vi "Main.vi"(8 "Error In":errorcluster, 11 "Simulate hardware?":bool) -> (0 "Error Out":errorcluster)   [LabVIEW 2017, in "DAQ.lvlib"]
uses:
  DAQ.lvlib
  Controls/Commands [enum].ctl
  Controls/Params.ctl
  Controls/DAQ Config.ctl
  Controls/DAQ Indicators.ctl
  System Control/CTLs/Test Type.ctl
  File IO/Controls/Params.ctl
  Events/Controls/Action Refs [enum].ctl
  Background Level Global.vi
  System Control/Main controller.lvlib
  Events/Events.lvlib
  File IO/File IO.lvlib
  UI/UI.lvlib
panel:
  out "Indicators":T1={"Data"={"Live"={"t0"=timestamp(0 s since 1904-01-01), "dt"=1.0, "Y"=[]}, "Accumulated"={"t0"=timestamp(0 s since 1904-01-01), "dt"=1.0, "Y"=[]}, "Averaged"={"t0"=timestamp(0 s since 1904-01-01), "dt"=1.0, "Y"=[]}, "data array"=[], "live time array"=[], "Live (decimated)"={"t0"=timestamp(0 s since 1904-01-01), "dt"=1.0, "Y"=[]}}, "Config"={"Input Config"=-1, "Card"=enum."USB-6211", "100% Reflectance Standard (V)"=1.0, "Input Channel"="", "Average number of points"=50.0, "Trigger Level (V)"=0.2, "Rate (Hz)"=250000, "End Time (s)"=1.0}, "Indicators"={"Final number of points"=5500.0, "Number of samples"=275000.0, "dt"=4e-06, "Shots"=1, "Shot counter"=0, "Test counter"=0, "Background level (V)"=0.0, "DAQ task"="", "timestamp of data"=timestamp(0 s since 1904-01-01), "Test Type"=enum."A-Test"}} {"Config"."Input Config" items=["default"=-1, "RSE"=10083, "NRSE"=10078, "Differential"=10106, "Pseudodifferential"=12529]}
  in  "File IO parameters - DEBUG":T5={"Output Folder"=path "C:/Users/Abigail/Documents/Imperial Optical software/Optical Software Code Simplified/Output", "Error file"=path "Error Log.txt", "Config file"=path "Config.ini", "File prefix"="600 nm", "Waveform read"={"t0"=timestamp(0 s since 1904-01-01), "dt"=1.0, "Y"=[]}}
  out "Live data incl. pre-trigger":cluster{"live time array":dbl[], "Y":dbl[]}(graph)
  out "Live data (cropped)":dbl[](graph)
  out "Accumulated data":waveform(dbl)(graph)={"t0"=timestamp(3604915966.0623617 s since 1904-01-01), "dt"=0.00019999999999999998, "Y"=[]}
  out "Averaged data":waveform(dbl)(graph)={"t0"=timestamp(3604915977.982374 s since 1904-01-01), "dt"=0.00019999999999999998, "Y"=[]}
  in  "Config In":T1={"Data"={"Live"={"t0"=timestamp(0 s since 1904-01-01), "dt"=1.0, "Y"=[]}, "Accumulated"={"t0"=timestamp(0 s since 1904-01-01), "dt"=1.0, "Y"=[]}, "Averaged"={"t0"=timestamp(0 s since 1904-01-01), "dt"=1.0, "Y"=[]}, "data array"=[], "live time array"=[], "Live (decimated)"={"t0"=timestamp(0 s since 1904-01-01), "dt"=1.0, "Y"=[]}}, "Config"={"Input Config"=-1, "Card"=enum."USB-6211", "100% Reflectance Standard (V)"=1.0, "Input Channel"="", "Average number of points"=50.0, "Trigger Level (V)"=0.2, "Rate (Hz)"=250000, "End Time (s)"=1.0}, "Indicators"={"Final number of points"=5500.0, "Number of samples"=275000.0, "dt"=4e-06, "Shots"=1, "Shot counter"=0, "Test counter"=0, "Background level (V)"=0.0, "DAQ task"="", "timestamp of data"=timestamp(0 s since 1904-01-01), "Test Type"=enum."A-Test"}} {"Config"."Input Config" items=["default"=-1, "RSE"=10083, "NRSE"=10078, "Differential"=10106, "Pseudodifferential"=12529]}
  in  "Set state":T6
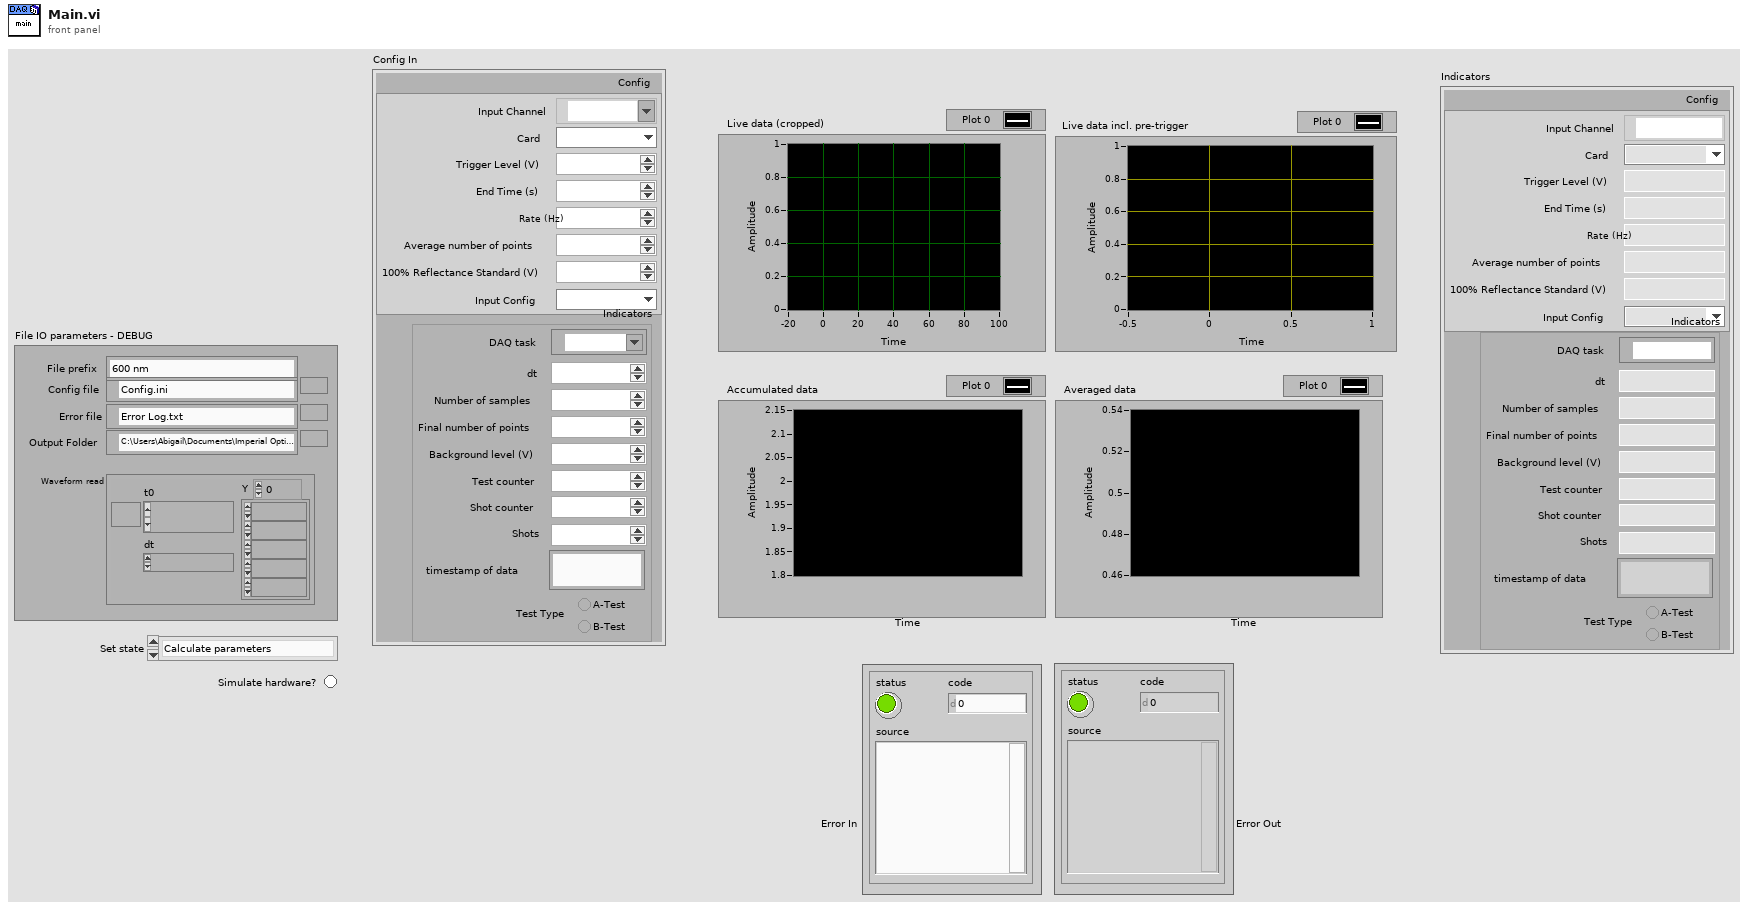
[diagram p1: front panel]
types:
  T1 = typedef "DAQ.lvlib/Params.ctl" = cluster{"Data":cluster{"Live":waveform(dbl), "Accumulated":waveform(dbl), "Averaged":waveform(dbl), "data array":dbl[], "live time array":dbl[], "Live (decimated)":waveform(dbl)}, "Config":T2, "Indicators":T3}
  T2 = typedef "DAQ.lvlib/DAQ Config.ctl" = cluster{"Input Config":i32, "Card":enum16{"USB-6211", "USB-6251", "USB-6361"}, "100% Reflectance Standard (V)":dbl, "Input Channel":tag, "Average number of points":dbl, "Trigger Level (V)":dbl, "Rate (Hz)":i32, "End Time (s)":dbl}
  T3 = typedef "DAQ.lvlib/DAQ Indicators.ctl" = cluster{"Final number of points":dbl, "Number of samples":dbl, "dt":dbl, "Shots":i32, "Shot counter":i32, "Test counter":i32, "Background level (V)":dbl, "DAQ task":refnum<k21>, "timestamp of data":timestamp, "Test Type":T4}
  T4 = typedef "Main controller.lvlib/Test Type.ctl" = enum32{"A-Test", "B-Test"}
  T5 = typedef "File IO.lvlib/Params.ctl" = cluster{"Output Folder":path, "Error file":path, "Config file":path, "File prefix":string, "Waveform read":waveform(dbl)}
  T6 = typedef "DAQ.lvlib/Commands [enum].ctl" = enum16{"Calculate parameters", "Start", "Stop", "Get test data", "Accumulate test data", "Average test data", "Calculate background voltage", "Send data", "Write data to file"}
  T7 = enum32{"Bad", "Idle", "Run top level", "Running"}
  T8 = typedef "Events.lvlib/Action Refs [enum].ctl" = enum16{"Init", "Ref", "Kill"}
  T9 = typedef "Events.lvlib/Refs [cluster].ctl" = cluster{"Exit":refnum<user-event>, "Controller":refnum<user-event>, "System Error":refnum<user-event>, "UI":refnum<user-event>, "Example Module":refnum<user-event>, "Shutter":refnum<user-event>, "Monochromator":refnum<user-event>, "DAQ":refnum<user-event>, "Scope":refnum<user-event>, "Processing":refnum<user-event>, "File IO":refnum<user-event>, "Colour wheel":refnum<user-event>}
  T10 = cluster{"Live":waveform(dbl), "Accumulated":waveform(dbl), "Averaged":waveform(dbl), "data array":dbl[], "live time array":dbl[], "Live (decimated)":waveform(dbl)}
  T11 = cluster{"Waveform Data":dbl[][], "Waveform Name":string}
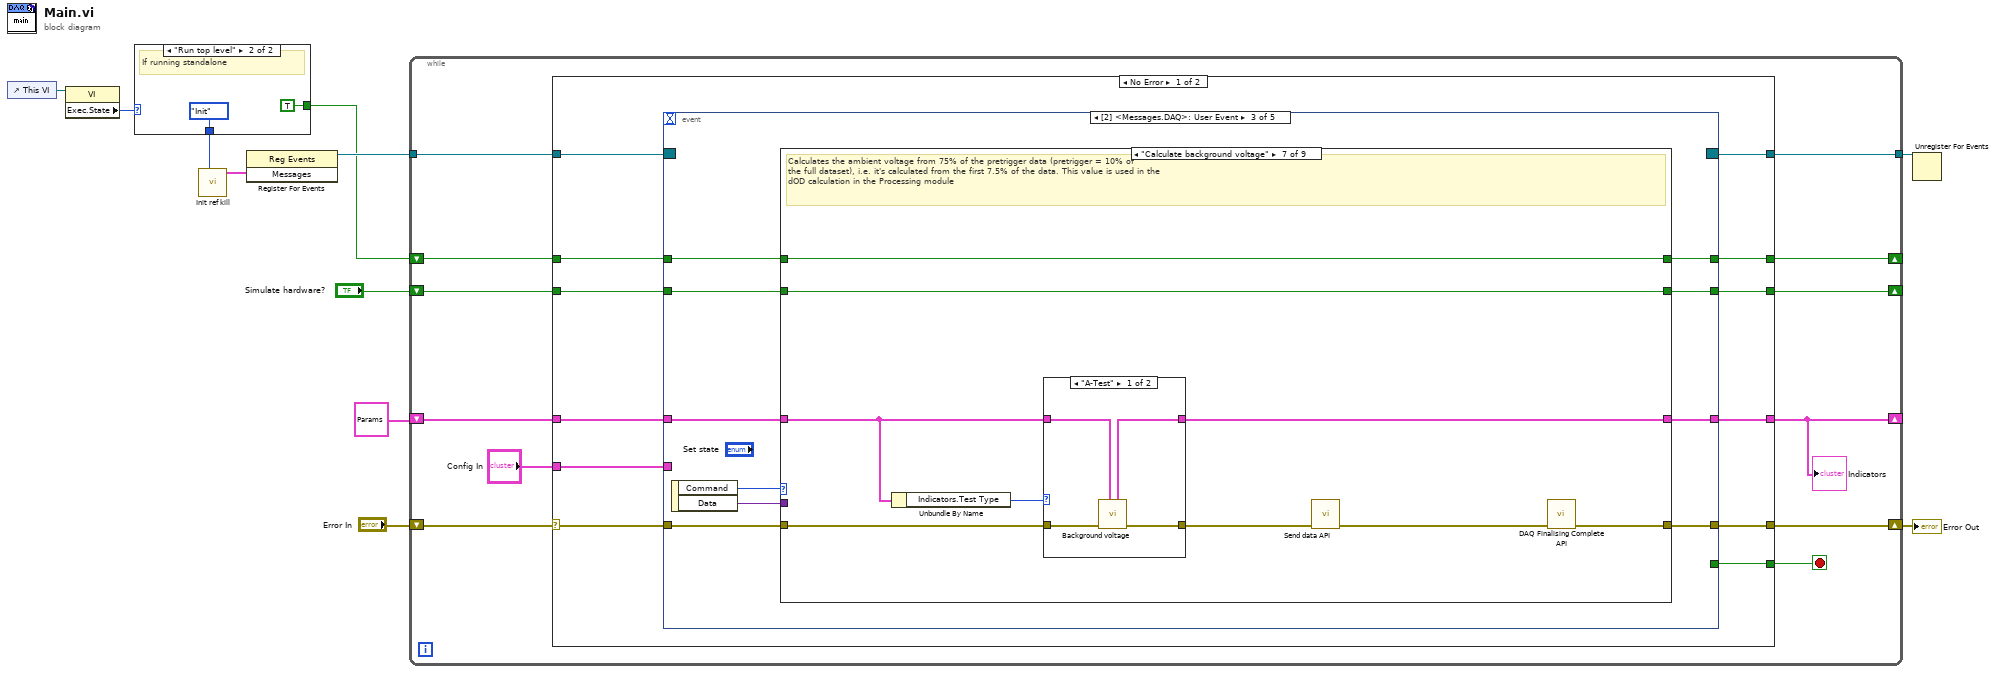
[diagram p0: block diagram]
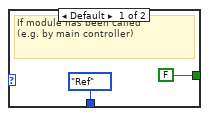
[diagram p2: hidden frame]
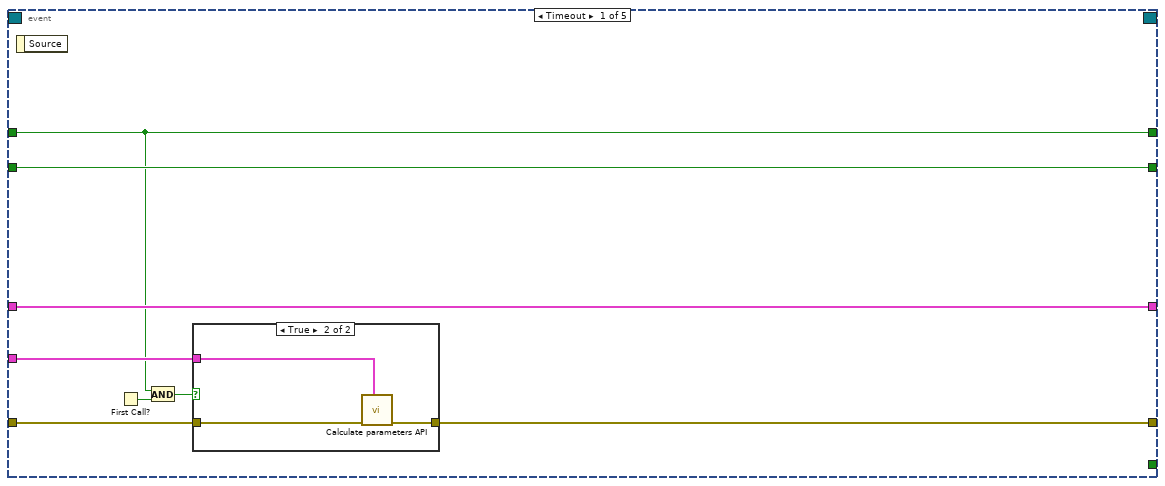
[diagram p3: hidden frame]
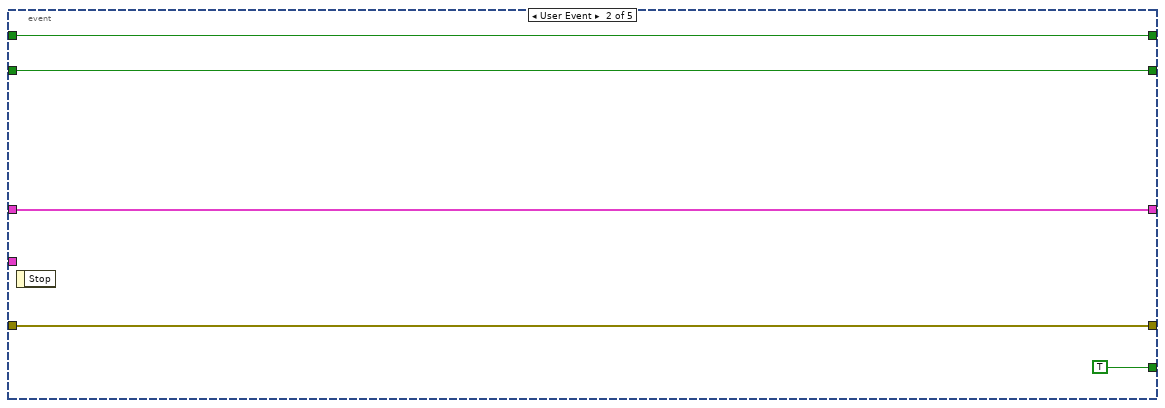
[diagram p5: hidden frame]
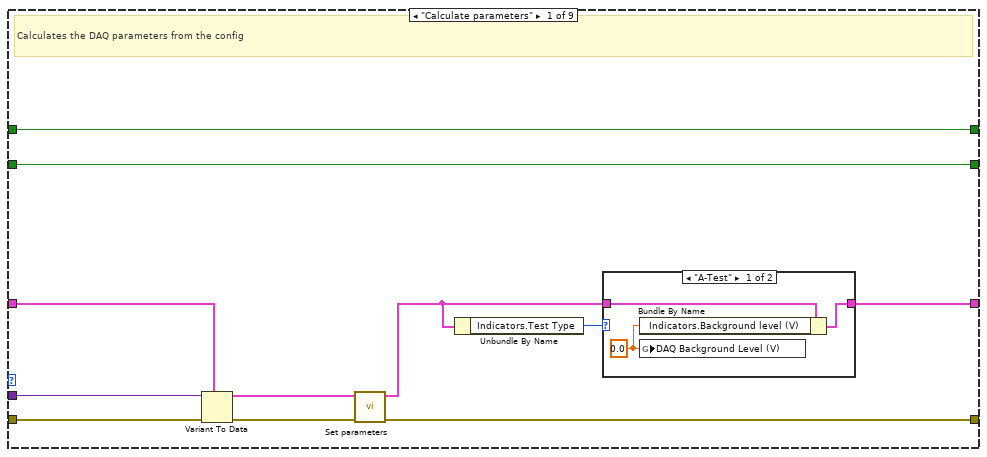
[diagram p6: hidden frame]
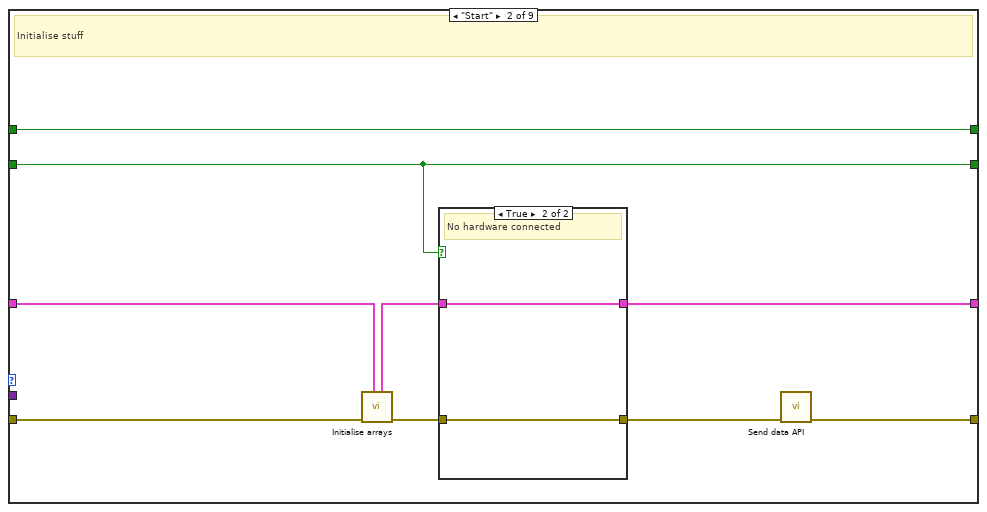
[diagram p8: hidden frame]
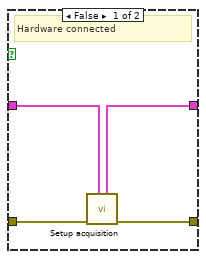
[diagram p9: hidden frame]
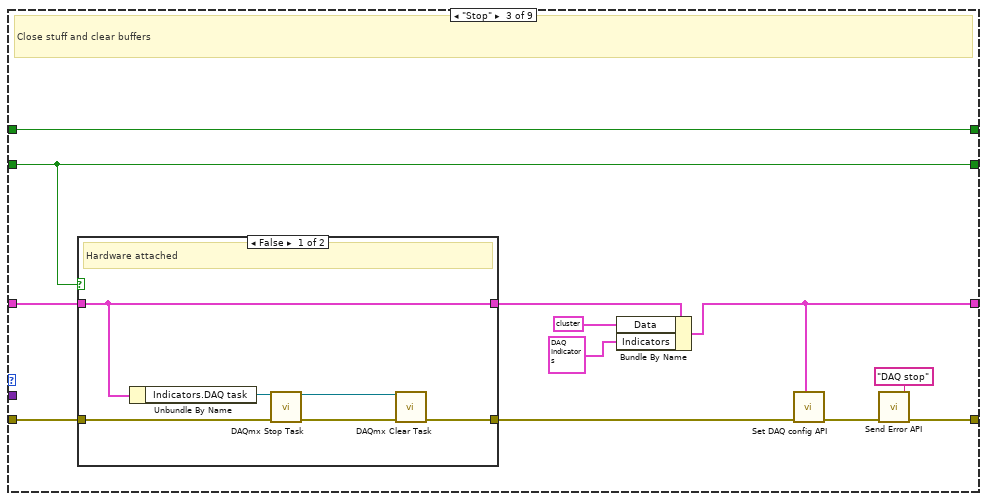
[diagram p10: hidden frame]
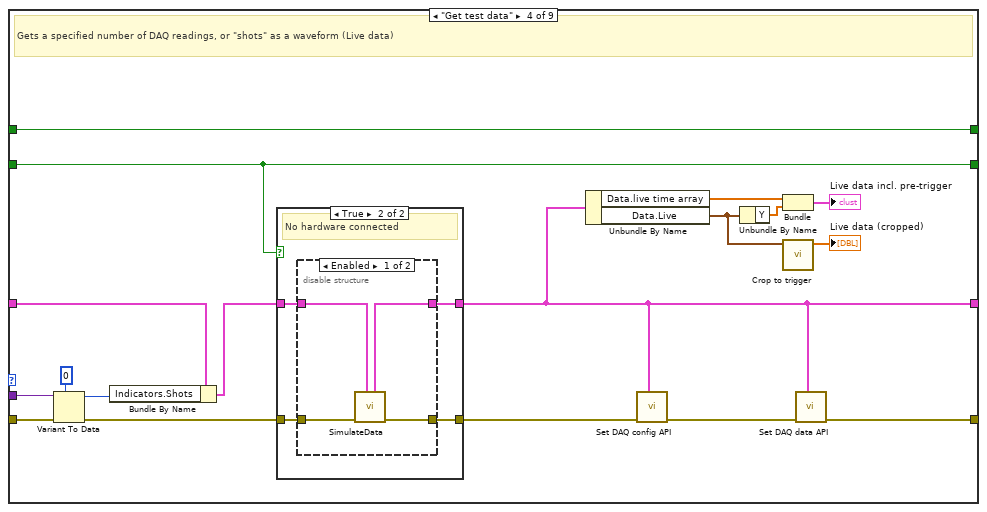
[diagram p12: hidden frame]
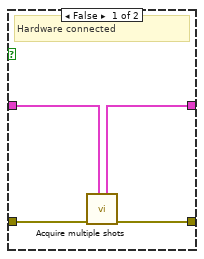
[diagram p13: hidden frame]
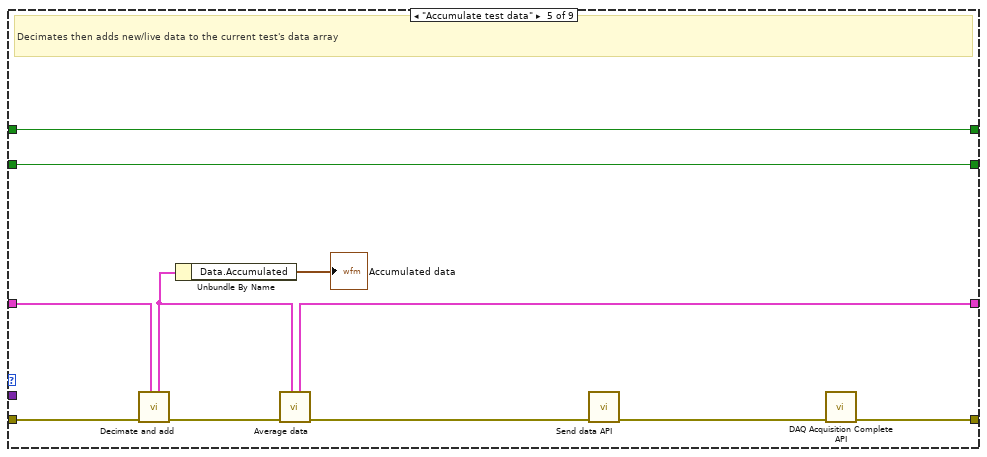
[diagram p15: hidden frame]
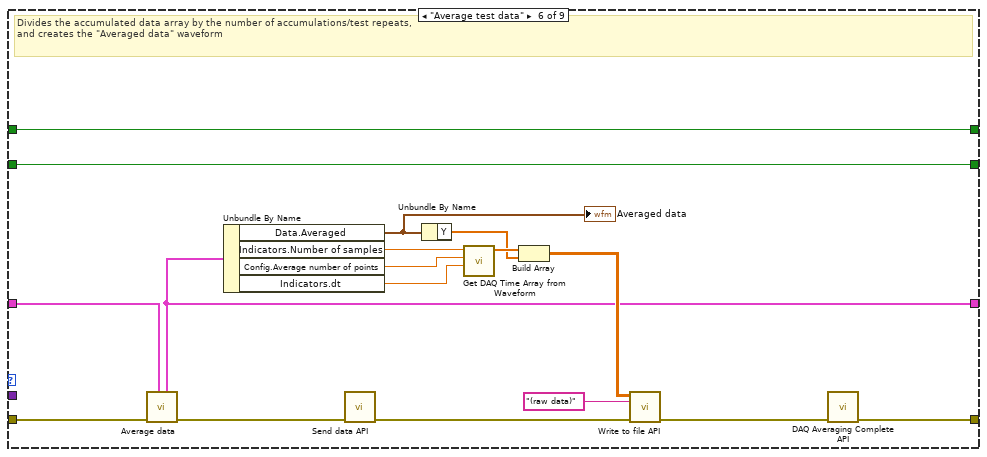
[diagram p16: hidden frame]
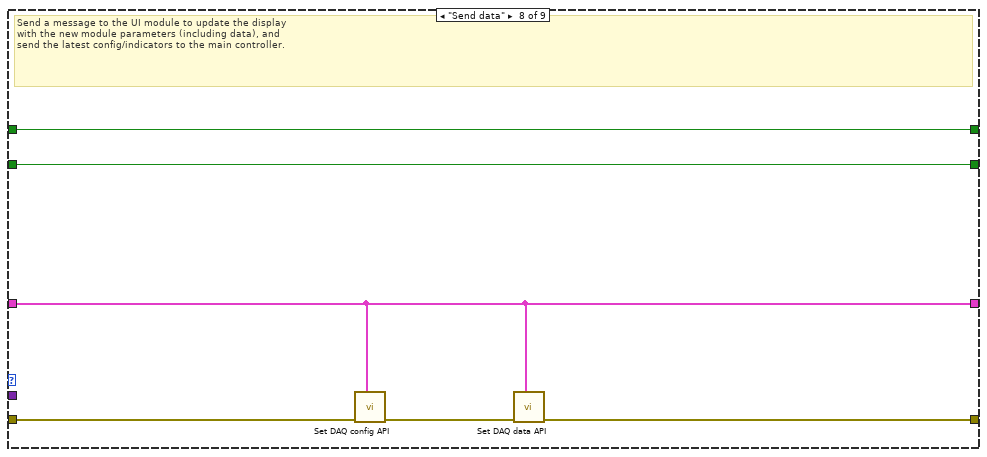
[diagram p18: hidden frame]
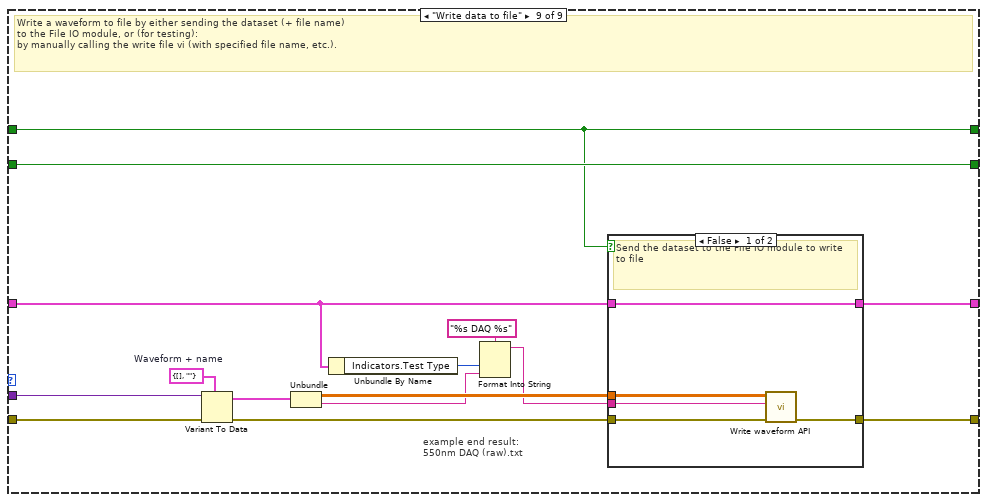
[diagram p19: hidden frame]
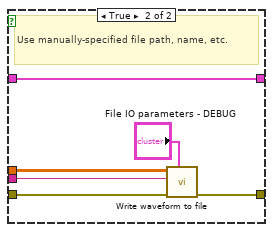
[diagram p20: hidden frame]
diagram:
  n1 = control-ref of="This VI"() -> (w6:refnum<vi>)
  n2 = property class="VI"(reference=w6) -> ("Exec.State"=w5:T7)  [unwired: 1 in, 2 out]
  n3 = case shown="\"Run top level\"" w5 {
    tunnel: [Action_Refs_[enum]."Ref" ("Action") Action_Refs_[enum]."Init" ("Action")] -> w4
    tunnel: [FALSE TRUE] -> w3
    frame Default {
      # "If module has been called\n(e.g. by main controller)"
    }
    frame "Run top level" {
      # "If running standalone"
    }
  }
  n4 = call "Init ref kill.vi"("Action"=w4) -> ("Messages"=w11:T9)  [unwired: 9 in, 1 out]
  n5 = register-events(w11) -> (reference out=w10:refnum<event-registration>)  [unwired: 2 in, 1 out]
  n6 = while {
    tunnel: w10 -> [w27]
    shift-right: [w24] -> _
    shift-left: "Simulate hardware?" -> [w23]
    tunnel: [w25] -> w9
    shift-right: [w21] -> w7
    shift-left: "Error In" -> [w20]
    shift-right: [w16] -> _
    shift-left: T1 {"Data"={"Live"={"t0"=timestamp(0 s since 1904-01-01), "dt"=1.0, "Y"=[]}, "Accumulated"={"t0"=timestamp(0 s since 1904-01-01), "dt"=1.0, "Y"=[]}, "Averaged"={"t0"=timestamp(0 s since 1904-01-01), "dt"=1.0, "Y"=[]}, "data array"=[], "live time array"=[], "Live (decimated)"={"t0"=timestamp(0 s since 1904-01-01), "dt"=1.0, "Y"=[]}}, "Config"={"Input Config"=-1, "Card"=enum."USB-6211", "100% Reflectance Standard (V)"=1.0, "Input Channel"="", "Average number of points"=50.0, "Trigger Level (V)"=0.2, "Rate (Hz)"=250000, "End Time (s)"=1.0}, "Indicators"={"Final number of points"=0.0, "Number of samples"=0.0, "dt"=0.0, "Shots"=1, "Shot counter"=0, "Test counter"=0, "Background level (V)"=0.0, "DAQ task"="", "timestamp of data"=timestamp(0 s since 1904-01-01), "Test Type"=enum."A-Test"}} ("Config 2") -> [w22]
    shift-right: [w18] -> _
    shift-left: w3 -> [w19]
    stop <- w26 stop-if-true
    n7 = case shown="No Error" w20 {
      selector: w20 -> [w31 w277]
      tunnel: w27 -> [w39 w273]
      tunnel: [w38 _] -> w26
      tunnel: [w37 w273] -> w25
      tunnel: [w36 w275] -> w24
      tunnel: w23 -> [w35 w275]
      tunnel: w22 -> [w34 w272]
      tunnel: [w33 w272] -> w16
      tunnel: [w32 w276] -> w21
      tunnel: w19 -> [w30 w274]
      tunnel: [w29 w274] -> w18
      tunnel: "Config In" -> [w28 _]
      frame No Error {
        n8 = event shown="[2] <Messages.DAQ>: User Event" {
          selector: w39 -> [_ _ _ _ _]
          dyn-events: [_ _ _ _ _] -> w37
          timeout: _ -> [_ _ _ _ _]
          tunnel: [_ TRUE _ _ _] -> w38
          tunnel: [w47 w53 w65 w228 w235] -> w36
          tunnel: w35 -> [w47 w53 w64 w228 w235]
          tunnel: w31 -> [w46 w54 w62 w226 w231]
          tunnel: [w45 w54 w61 w225 w230] -> w32
          tunnel: w34 -> [w44 w55 w60 _ w233]
          tunnel: [w44 w55 w59 w224 w232] -> w33
          tunnel: w30 -> [w42 w52 w57 w227 w229]
          tunnel: [w42 w52 w58 w227 w229] -> w29
          tunnel: w28 -> [w43 _ _ _ _]
          event Timeout {
            n9 = event-data() -> ()  [unwired: 1 in, 1 out]
            n10 = First Call?() -> (First Call?: T/F=w41:bool)
            n11 = And(x=w42, y=w41) -> (x .and. y?=w40:bool)
            n12 = case shown="True" w40 {
              tunnel: w46 -> [w48 w51]
              tunnel: [w48 w50] -> w45
              tunnel: w43 -> [_ w49]
              frame False {
              }
              frame True {
                n13 = call "Calculate parameters API.vi"("DAQ"=w49, "Error In"=w51) -> ("Error Out"=w50:errorcluster)  [unwired: 9 in]
              }
            }
          }
          event User Event {
            n14 = event-data() -> ()  [unwired: 1 in, 1 out]
          }
          event User Event {
            n15 = event-data() -> ("Command"=w66:T6, "Data"=w63:variant)  [unwired: 1 in]
            n16 = case shown="\"Calculate background voltage\"" w66 {
              tunnel: [w72 w89 w103 w131 w158 w175 w185 w197 w212] -> w65
              tunnel: w64 -> [w72 w89 w103 w131 w158 w175 w185 w197 w212]
              tunnel: w63 -> [w76 _ _ w125 _ _ _ _ w206]
              tunnel: w62 -> [w77 w86 w104 w127 w159 w176 w184 w196 w207]
              tunnel: [w71 w82 w108 w118 w154 w169 w182 w192 w203] -> w61
              tunnel: w60 -> [w75 w85 w105 w123 w155 w171 w178 w193 w200]
              tunnel: [w69 w84 w97 w117 w149 w162 w181 w193 w204] -> w59
              tunnel: [w73 w90 w106 w132 w157 w174 w183 w194 w205] -> w58
              tunnel: w57 -> [w73 w90 w106 w132 w157 w174 w183 w194 w205]
              frame "Calculate parameters" {
                # "Calculates the DAQ parameters from the config"
                n17 = Variant To Data(error in=w77, type=w75, Variant=w76) -> (data=w70:T1, error out=w74:errorcluster)
                n18 = call "Set parameters.vi"("error in"=w74, "DAQ"=w70) -> ("error out"=w71:errorcluster, "DAQ out"=w68:T1)  [unwired: 8 in]
                n19 = Unbundle By Name(w68) -> ("Indicators.Test Type"=w67:T4)
                n20 = case shown="\"A-Test\"" w67 {
                  tunnel: w68 -> [w80 w81]
                  tunnel: [w79 w81] -> w69
                  frame "A-Test" {
                    w78 = 0.0 ("DAQ Background Level (V)")
                    n21 = Bundle By Name(cluster=w80, "Indicators.Background level (V)"=w78) -> (w79:T1)
                    n22 = global write "Background Level Global.vi" "DAQ Background Level (V)"(w78) -> ()
                  }
                  frame "B-Test" {
                  }
                }
              }
              frame "Start" {
                # "Initialise stuff"
                n23 = call "Initialise arrays.vi"("DAQ"=w85, "error in"=w86) -> ("error out"=w88:errorcluster, "DAQ out"=w87:T1)  [unwired: 8 in]
                n24 = case shown="True" w89 {
                  tunnel: w88 -> [w94 w96]
                  tunnel: [w93 w96] -> w83
                  tunnel: [w92 w95] -> w84
                  tunnel: w87 -> [w91 w95]
                  frame False {
                    # "Hardware connected"
                    n25 = call "Setup acquisition.vi"("DAQ"=w91, "error in"=w94) -> ("error out"=w93:errorcluster, "DAQ out"=w92:T1)  [unwired: 8 in]
                  }
                  frame True {
                    # "No hardware connected"
                  }
                }
                n26 = call "Send data API.vi"("Error In"=w83) -> ("Error Out"=w82:errorcluster)  [unwired: 10 in]
              }
              frame "Stop" {
                # "Close stuff and clear buffers"
                n27 = case shown="False" w103 {
                  tunnel: w105 -> [w109 w116]
                  tunnel: w104 -> [w113 w115]
                  tunnel: [w112 w115] -> w99
                  tunnel: [w109 w116] -> w102
                  frame False {
                    # "Hardware attached"
                    n28 = Unbundle By Name(w109) -> ("Indicators.DAQ task"=w110:refnum<k21>)
                    n29 = call <vilib>:"DAQmx Stop Task.vi"("task/channels in"=w110, "error in"=w113) -> ("task out"=w114:refnum<k21>, "error out"=w111:errorcluster)  [unwired: 12 in]
                    n30 = call <vilib>:"DAQmx Clear Task.vi"("task in"=w114, "error in"=w111) -> ("error out"=w112:errorcluster)  [unwired: 13 in]
                  }
                  frame True {
                    # "No hardware attached"
                  }
                }
                n31 = Bundle By Name(cluster=w102, "Data"=T10 {"Live"={"t0"=timestamp(0 s since 1904-01-01), "dt"=1.0, "Y"=[]}, "Accumulated"={"t0"=timestamp(0 s since 1904-01-01), "dt"=1.0, "Y"=[]}, "Averaged"={"t0"=timestamp(0 s since 1904-01-01), "dt"=1.0, "Y"=[]}, "data array"=[], "live time array"=[], "Live (decimated)"={"t0"=timestamp(0 s since 1904-01-01), "dt"=1.0, "Y"=[]}}, "Indicators"=T3 {"Final number of points"=0.0, "Number of samples"=0.0, "dt"=0.0, "Shots"=0, "Shot counter"=0, "Test counter"=0, "Background level (V)"=0.0, "DAQ task"="", "timestamp of data"=timestamp(0 s since 1904-01-01), "Test Type"=enum."A-Test"}) -> (w97:T1)
                n32 = call "Set DAQ config API.vi"("DAQ config"=w97, "Error In"=w99) -> ("Error Out"=w98:errorcluster)  [unwired: 9 in]
                n33 = call "Send Error API.vi"("Error Cluster"=w98, "Error"="DAQ stop") -> ("Error Out"=w108:errorcluster)  [unwired: 9 in]
              }
              frame "Get test data" {
                # "Gets a specified number of DAQ readings, or \"shots\" as a waveform (Live data)"
                n34 = Variant To Data(error in=w127, type=0, Variant=w125) -> (data=w124:i32, error out=w126:errorcluster)
                n35 = Bundle By Name(cluster=w123, "Indicators.Shots"=w124) -> (w122:T1)
                n36 = case shown="True" w131 {
                  tunnel: w126 -> [w138 w142]
                  tunnel: [w137 w141] -> w119
                  tunnel: [w136 w140] -> w117
                  tunnel: w122 -> [w135 w139]
                  frame False {
                    # "Hardware connected"
                    n37 = call "Acquire multiple shots.vi"("DAQ"=w135, "error in (no error)"=w138) -> ("error out"=w137:errorcluster, "DAQ out"=w136:T1)  [unwired: 8 in]
                  }
                  frame True {
                    # "No hardware connected"
                    n38 = disable-structure shown="Enabled" {
                      disable-tunnel: w142 -> [w146 w147]
                      disable-tunnel: [w145 w147] -> w141
                      disable-tunnel: [w144 w148] -> w140
                      disable-tunnel: w139 -> [w143 w148]
                      frame Enabled {
                        n39 = call "SimulateData.vi"("DAQ"=w143, "error in (no error)"=w146) -> ("error out"=w145:errorcluster, "DAQ out"=w144:T1)  [unwired: 8 in]
                      }
                      frame Disabled {
                      }
                    }
                  }
                }
                n40 = Unbundle By Name(w117) -> ("Data.live time array"=w133:dbl[], "Data.Live"=w128:waveform(dbl))
                n41 = call "Set DAQ config API.vi"("DAQ config"=w117, "Error In"=w119) -> ("Error Out"=w120:errorcluster)  [unwired: 9 in]
                n42 = Unbundle By Name(w128) -> ("Y"=w130:dbl[])
                n43 = Bundle("live time array"=w133, "Y"=w130) -> (→"Live data incl. pre-trigger":cluster{"live time array":dbl[], "Y":dbl[]})  [unwired: 1 in]
                n44 = call "Crop to trigger.vi"("Live"=w128) -> ("Live data"=→"Live data (cropped)":dbl[])  [unwired: 10 in]
                n45 = call "Set DAQ data API.vi"("Config"=w117, "Error In"=w120) -> ("Error Out"=w118:errorcluster)  [unwired: 9 in]
              }
              frame "Accumulate test data" {
                # "Decimates then adds new/live data to the current test's data array"
                n46 = call "Decimate and add.vi"("DAQ"=w155, "error in"=w159) -> ("error out"=w152:errorcluster, "DAQ out"=w150:T1)  [unwired: 7 in, 1 out]
                n47 = Unbundle By Name(w150) -> ("Data.Accumulated"=→"Accumulated data":waveform(dbl))
                n48 = call "Average data.vi"("DAQ In"=w150, "error in"=w152) -> ("error out"=w151:errorcluster, "DAQ out"=w149:T1)  [unwired: 8 in]
                n49 = call "Send data API.vi"("Error In"=w151) -> ("Error Out"=w153:errorcluster)  [unwired: 10 in]
                n50 = call "DAQ Acquisition Complete API.vi"("Error In"=w153) -> ("Error Out"=w154:errorcluster)  [unwired: 10 in]
              }
              frame "Average test data" {
                # "Divides the accumulated data array by the number of accumulations/test repeats, \nand creates the \"Averaged data\" waveform"
                n51 = call "Average data.vi"("DAQ In"=w171, "error in"=w176) -> ("error out"=w161:errorcluster, "DAQ out"=w162:T1)  [unwired: 8 in]
                n52 = Unbundle By Name(w162) -> ("Data.Averaged"=w173:waveform(dbl), "Indicators.Number of samples"=w168:dbl, "Config.Average number of points"=w167:dbl, "Indicators.dt"=w163:dbl)
                "Averaged data" <- w173
                n53 = call "Send data API.vi"("Error In"=w161) -> ("Error Out"=w160:errorcluster)  [unwired: 10 in]
                n54 = Unbundle By Name(w173) -> ("Y"=w165:dbl[])
                n55 = call "Get DAQ Time Array from Waveform.vi"("DAQ dt"=w163, "DAQ Average Number of Points"=w167, "DAQ Number of Samples"=w168) -> ("Time Axis"=w166:dbl[])  [unwired: 7 in, 1 out]
                n56 = Build Array(w166, w165) -> (w164:dbl[][])
                n57 = call "Write to file API.vi"("Error In"=w160, "Waveform name"="(raw data)" ("DAQ average file"), "Waveform Data"=w164) -> ("Error Out"=w170:errorcluster)  [unwired: 8 in]
                n58 = call "DAQ Averaging Complete API.vi"("Error In"=w170) -> ("Error Out"=w169:errorcluster)  [unwired: 10 in]
              }
              frame "Calculate background voltage" {
                # "Calculates the ambient voltage from 75% of the pretrigger data (pretrigger = 10% of \nthe full dataset), i.e. it's calculated from the first 7.5% of the data. This value is used in the \ndOD calculation in the Processing module"
                n59 = Unbundle By Name(w178) -> ("Indicators.Test Type"=w177:T4)
                n60 = case shown="\"A-Test\"" w177 {
                  tunnel: w184 -> [w189 w190]
                  tunnel: [w188 w191] -> w181
                  tunnel: [w187 w190] -> w180
                  tunnel: w178 -> [w186 w191]
                  frame "A-Test" {
                    n61 = call "Background voltage.vi"("DAQ"=w186, "error in"=w189) -> ("error out"=w187:errorcluster, "DAQ out"=w188:T1)  [unwired: 8 in]
                  }
                  frame "B-Test" {
                  }
                }
                n62 = call "Send data API.vi"("Error In"=w180) -> ("Error Out"=w179:errorcluster)  [unwired: 10 in]
                n63 = call "DAQ Finalising Complete API.vi"("Error In"=w179) -> ("Error Out"=w182:errorcluster)  [unwired: 10 in]
              }
              frame "Send data" {
                # "Send a message to the UI module to update the display \nwith the new module parameters (including data), and \nsend the latest config/indicators to the main controller."
                n64 = call "Set DAQ config API.vi"("DAQ config"=w193, "Error In"=w196) -> ("Error Out"=w195:errorcluster)  [unwired: 9 in]
                n65 = call "Set DAQ data API.vi"("Config"=w193, "Error In"=w195) -> ("Error Out"=w192:errorcluster)  [unwired: 9 in]
              }
              frame "Write data to file" {
                w211 = T11 {"Waveform Data"=[], "Waveform Name"=""}  # Waveform + name
                # "example end result:\n550nm DAQ (raw).txt"
                # "Write a waveform to file by either sending the dataset (+ file name) \nto the File IO module, or (for testing):\nby manually calling the write file vi (with specified file name, etc.)."
                n66 = Variant To Data(error in=w207, type=w211, Variant=w206) -> (data=w208:T11, error out=w209:errorcluster)
                n67 = Unbundle(w208) -> ("Waveform Data"=w210:dbl[][], "Waveform Name"=w199:string)
                n68 = Unbundle By Name(w200) -> ("Indicators.Test Type"=w201:T4)
                n69 = Format Into String(format string="%s DAQ %s", w201, w199) -> (resulting string=w198:string)  [unwired: 2 in, 1 out]
                n70 = case shown="False" w205 {
                  tunnel: [w217 w223] -> w203
                  tunnel: w210 -> [w216 w222]
                  tunnel: w209 -> [w215 w221]
                  tunnel: w198 -> [w214 w220]
                  tunnel: [w213 w219] -> w204
                  tunnel: w200 -> [w213 w219]
                  frame False {
                    # "Send the dataset to the File IO module to write to file"
                    n71 = call "Write waveform API.vi"("Error In"=w215, "Waveform name"=w214, "Waveform Data"=w216) -> ("Error Out"=w217:errorcluster)  [unwired: 8 in]
                  }
                  frame True {
                    # "Use manually-specified file path, name, etc."
                    n72 = call "Write waveform to file.vi"("File IO parameters"="File IO parameters - DEBUG", "error in"=w221, "Dataset name"=w220, "Data"=w222) -> ("error out"=w223:errorcluster)  [unwired: 7 in]
                  }
                }
              }
            }
          }
          event Value Change {
            n73 = event-data() -> ("NewVal"=w224:T1)  [unwired: 1 in]
            n74 = call "Calculate parameters API.vi"("DAQ"=w224, "Error In"=w226) -> ("Error Out"=w225:errorcluster)  [unwired: 9 in]
          }
          event Value Change {
            n75 = event-data() -> ("NewVal"=w234:T6)  [unwired: 1 in]
            n76 = case shown="\"Write data to file\"" w234 {
              tunnel: w233 -> [w238 w239 w244 w248 w251 w254 w257 w260 w262]
              tunnel: [w238 w239 w244 w248 w251 w254 w257 w260 w262] -> w232
              tunnel: [w236 w240 w242 w246 w249 w252 w255 w258 w270] -> w230
              tunnel: w231 -> [w237 w241 w243 w247 w250 w253 w256 w259 w271]
              frame "Calculate parameters" {
                n77 = call "Calculate parameters API.vi"("DAQ"=w238, "Error In"=w237) -> ("Error Out"=w236:errorcluster)  [unwired: 9 in]
              }
              frame "Start" {
                n78 = call "Start API.vi"("Error In"=w241) -> ("Error Out"=w240:errorcluster)  [unwired: 10 in]
              }
              frame "Stop" {
                n79 = call "Stop API.vi"("Error In"=w243) -> ("Error Out"=w242:errorcluster)  [unwired: 10 in]
              }
              frame "Get test data" {
                n80 = call "Get test data API.vi"("Error In"=w247, "Shots"=1) -> ("Error Out"=w246:errorcluster)  [unwired: 9 in]
              }
              frame "Accumulate test data" {
                n81 = call "Accumulate data API.vi"("Error In"=w250) -> ("Error Out"=w249:errorcluster)  [unwired: 10 in]
              }
              frame "Average test data" {
                n82 = call "Average data API.vi"("Error In"=w253) -> ("Error Out"=w252:errorcluster)  [unwired: 10 in]
              }
              frame "Calculate background voltage" {
                n83 = call "Background voltage API.vi"("Error In"=w256) -> ("Error Out"=w255:errorcluster)  [unwired: 10 in]
              }
              frame "Send data" {
                n84 = call "Send data API.vi"("Error In"=w259) -> ("Error Out"=w258:errorcluster)  [unwired: 10 in]
              }
              frame "Write data to file" {
                n85 = Unbundle By Name(w262) -> ("Data.Live"=w268:waveform(dbl), "Indicators.Number of samples"=w267:dbl, "Config.Average number of points"=w266:dbl)
                n86 = Unbundle By Name(w268) -> ("Y"=w263:dbl[], "dt"=w265:dbl)
                n87 = call "Get DAQ Time Array from Waveform.vi"("DAQ dt"=w265, "DAQ Average Number of Points"=w266, "DAQ Number of Samples"=w267) -> ("Time Axis"=w264:dbl[])  [unwired: 7 in, 1 out]
                n88 = Build Array(w264, w263) -> (w261:dbl[][])
                n89 = call "Write to file API.vi"("Error In"=w271, "Waveform name"="(raw)", "Waveform Data"=w261) -> ("Error Out"=w270:errorcluster)  [unwired: 8 in]
              }
            }
          }
        }
      }
      frame Error {
        n90 = case shown="True" w274 {
          tunnel: w277 -> [w279 w284]
          tunnel: [w278 _] -> w276
          frame False {
            n91 = case shown="Error" w279 {
              selector: w279 -> [w280 w282]
              tunnel: [w280 w283] -> w278
              frame No Error {
              }
              frame Error {
                n92 = call "Send Error API.vi"("Error Cluster"=w282) -> ("Error Out"=w281:errorcluster)  [unwired: 10 in]
                n93 = call "Log error API.vi"("Error In"=w281) -> ("Error Out"=w283:errorcluster)  [unwired: 10 in]
              }
            }
          }
          frame True {
            n94 = call <vilib>:"Simple Error Handler.vi"("error in (no error)"=w284) -> ()  [unwired: 4 in, 5 out]
          }
        }
      }
    }
    "Indicators" <- w16
  }
  "Error Out" <- w7
  n95 = Unregister For Events(event registration refnum=w9) -> ()  [unwired: 1 in, 1 out]
